vi "Get artiq-client command.vi"(9 "sub-command":string, 11 "Kasli Wrapper 2.0 in":refnum<class "Kasli Wrapper 2.0.lvclass">) -> (1 "command":string, 3 "Kasli Wrapper 2.0 out":refnum<class "Kasli Wrapper 2.0.lvclass">)   [LabVIEW 2020, in "CIRCUS_uServices.lvlib" / "Kasli Wrapper 2.0.lvlib" / "Kasli Wrapper 2.0.lvclass"]
uses:
  Kasli Wrapper 2.0.lvclass
  Kasli Wrapper 2.0.lvclass/Kasli Wrapper 2.0.ctl
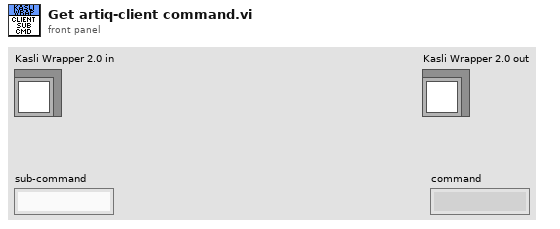
[diagram p1: front panel]
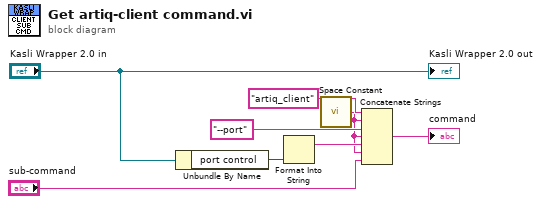
[diagram p0: block diagram]
diagram:
  n1 = Unbundle By Name("Kasli Wrapper 2.0 in") -> ("port control"=w5:u32)
  n2 = Format Into String(w5) -> (resulting string=w4:string)  [unwired: 3 in, 1 out]
  n3 = call <vilib>:"Space Constant.vi"() -> ("String"=w1:string)
  n4 = Concatenate Strings("artiq_client" ("standard input"), w1, "--port" ("initial string"), w1, w4, w1, "sub-command") -> (→"command":string)
  "Kasli Wrapper 2.0 out" <- "Kasli Wrapper 2.0 in"
